vi "get_trajectory.vi"(8 "error in (no error)":errorcluster, 11 "GenericScanHead.lvclass in":refnum<class "GenericScanHead.lvclass">) -> (0 "error out":errorcluster, 2 "trajectory":refnum<class "GenericTrajectory.lvclass">, 3 "GenericScanHead.lvclass out":refnum<class "GenericScanHead.lvclass">)   [LabVIEW 2010, in "GenericScanHead.lvclass"]
uses:
  GenericScanHead.lvclass
  Trajectory/GenericTrajectory/GenericTrajectory/GenericTrajectory.lvclass
  GenericScanHead.lvclass/GenericScanHead.ctl
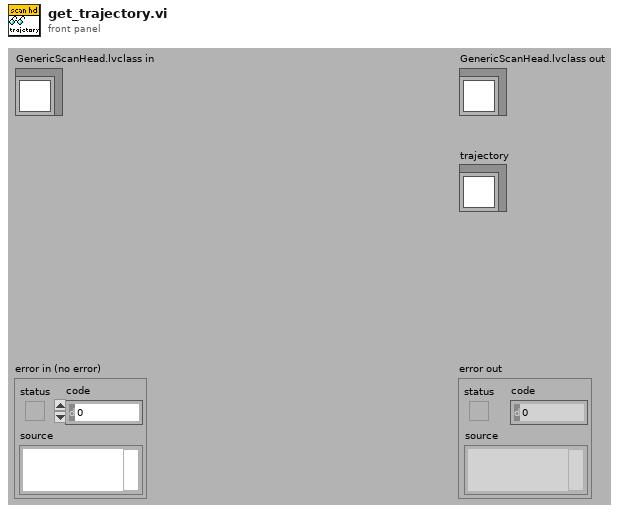
[diagram p1: front panel]
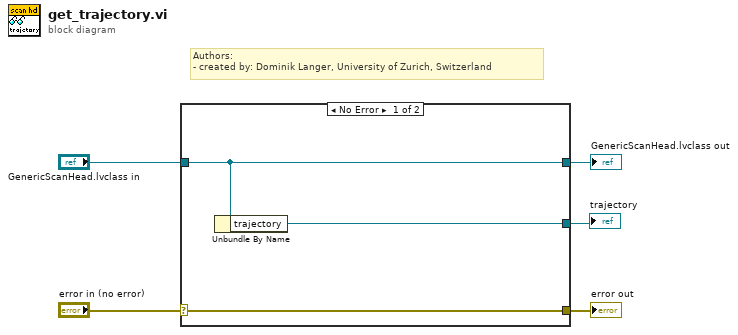
[diagram p0: block diagram]
diagram:
  # "Authors: \n- created by: Dominik Langer, University of Zurich, Switzerland"
  n1 = case shown="No Error" "error in (no error)" {
    selector: "error in (no error)" -> [w8 w9]
    tunnel: [w8 w9] -> w4
    tunnel: [w7 w10] -> w2
    tunnel: "GenericScanHead.lvclass in" -> [w7 w10]
    tunnel: [w6 _] -> w1
    frame No Error {
      n2 = Unbundle By Name(w7) -> ("trajectory"=w6:refnum<class "GenericTrajectory.lvclass">)
    }
    frame Error {
    }
  }
  "error out" <- w4
  "GenericScanHead.lvclass out" <- w2
  "trajectory" <- w1
